vi "CheckDeviceFCG.vi"() -> ()   [LabVIEW 2010]
panel:
  out "WavelenghtArrayOut":i32[](array[numeric])
  out "OnlineStatusLaserPower":bool
  out "Interlock":bool
  out "Diode (pump) current / [mA]":i32(knob)=2 scale=0.0..700.0
  out "Booster 1 current / [mA]":i32(knob) scale=0.0..5000.0
  out "Output photodiode current / [mA]":i32(knob) scale=0.0..200.0
  out "Actual Power Level / [%]":i8(knob) scale=0.0..100.0
  out "Temperature sensor 1 / [°C]":i8(knob)=24 scale=20.0..30.0
  out "Temperature sensor 3 / [°C]":i8(knob)=25 scale=20.0..30.0
  out "Temperature sensor 2 / [°C]":i8(knob)=24 scale=20.0..30.0
  out "Temperature sensor 0 / [°C]":i8(knob)=23 scale=20.0..30.0
  out "andorscanner":bool
  out "710 Get":bool
  out "517 Get":bool
  out "ctiotf Get":bool
  out "Camera Get":bool
  out "Seed Laser Get":bool caption="seed laser"
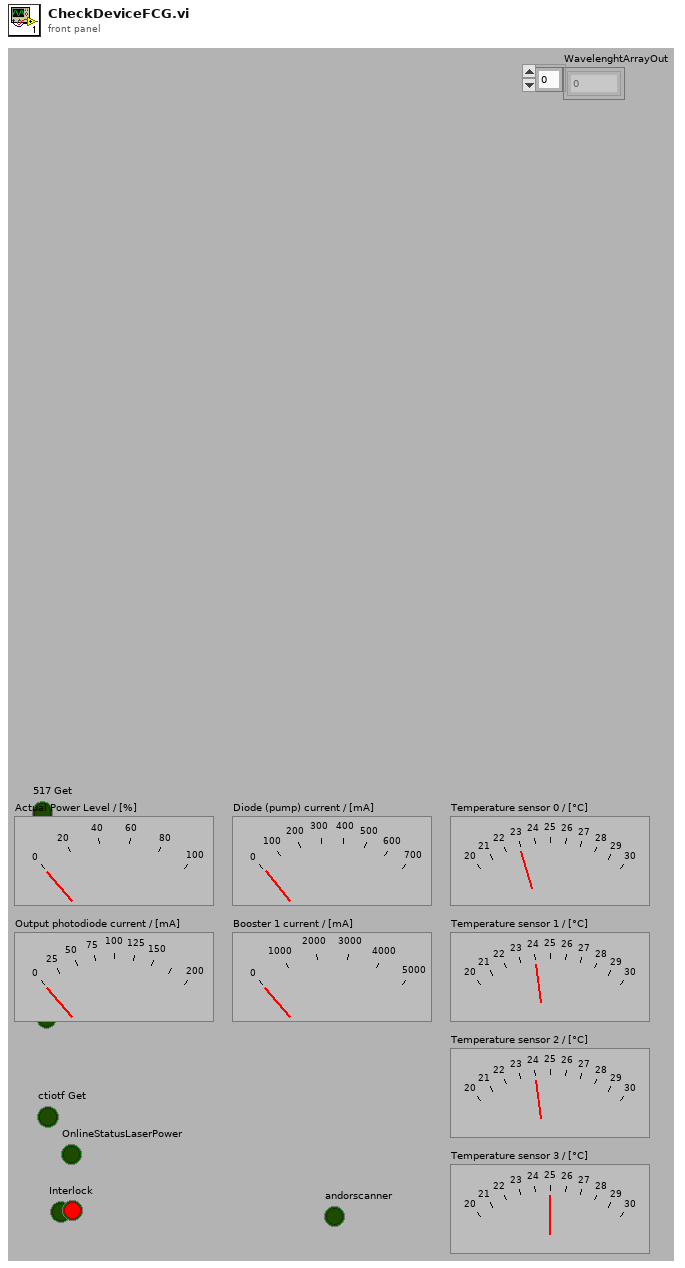
[diagram p1: front panel]
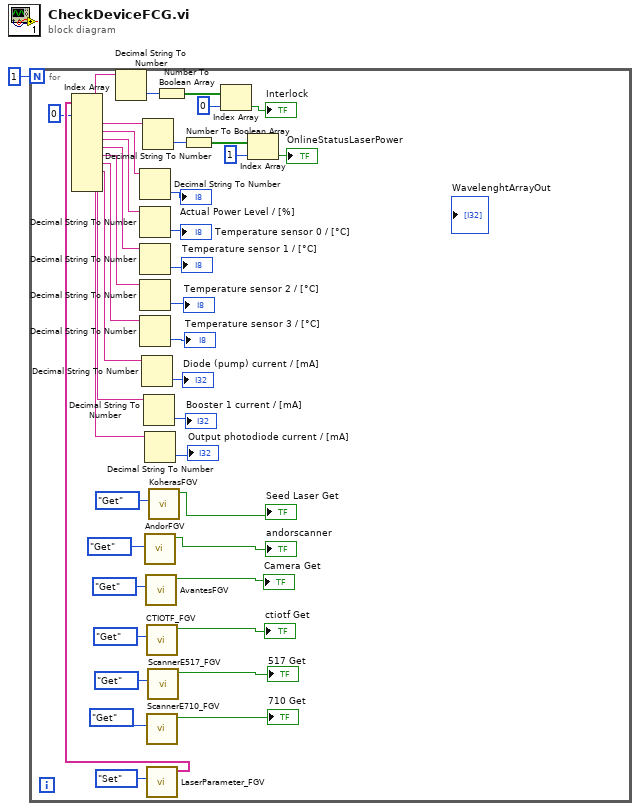
[diagram p0: block diagram]
diagram:
  n1 = for {
    N: 1 -> [_]
    n2 = call "AndorFGV.vi"("Set_Get"=enum16{"Set", "Get"}."Get") -> ("andor 0"=→"andorscanner":bool)  [unwired: 8 in, 2 out]
    n3 = call "AvantesFGV.vi"("Set_Get"=enum16{"Set", "Get"}."Get") -> ("Get"=→"Camera Get":bool)  [unwired: 9 in, 1 out]
    n4 = call "CTIOTF_FGV.vi"("Set_Get"=enum16{"Set", "Get"}."Get") -> ("aotfGet"=→"ctiotf Get":bool)  [unwired: 9 in, 1 out]
    n5 = call "ScannerE710_FGV.vi"("Set_Get"=enum16{"Set", "Get"}."Get") -> ("Get"=→"710 Get":bool)  [unwired: 9 in, 1 out]
    n6 = call "LaserParameter_FGV.vi"("Set_Get"=enum16{"Set", "Get"}."Set") -> ("LaserParameterGet"=w5:string[])  [unwired: 9 in, 1 out]
    n7 = Index Array(array=w5, index #1=0 ("index")) -> (element #1=w21:string, element #2=w20:string, element #3=w19:string, element #4=w18:string, element #5=w11:string, element #6=w10:string, element #7=w9:string, element #8=w8:string, element #9=w7:string, element #10=w6:string)  [unwired: 9 in]
    n8 = Decimal String To Number(string=w21) -> (number=w17:i32)  [unwired: 2 in, 1 out]
    n9 = Decimal String To Number(string=w19) -> (number=→"Actual Power Level / [%]":i32)  [unwired: 2 in, 1 out]
    n10 = Decimal String To Number(string=w18) -> (number=→"Temperature sensor 0 / [°C]":i32)  [unwired: 2 in, 1 out]
    n11 = Decimal String To Number(string=w11) -> (number=→"Temperature sensor 1 / [°C]":i32)  [unwired: 2 in, 1 out]
    n12 = Decimal String To Number(string=w10) -> (number=→"Temperature sensor 2 / [°C]":i32)  [unwired: 2 in, 1 out]
    n13 = Decimal String To Number(string=w9) -> (number=→"Temperature sensor 3 / [°C]":i32)  [unwired: 2 in, 1 out]
    n14 = Decimal String To Number(string=w8) -> (number=→"Diode (pump) current / [mA]":i32)  [unwired: 2 in, 1 out]
    n15 = Decimal String To Number(string=w20) -> (number=w16:i32)  [unwired: 2 in, 1 out]
    n16 = Decimal String To Number(string=w7) -> (number=→"Booster 1 current / [mA]":i32)  [unwired: 2 in, 1 out]
    n17 = Decimal String To Number(string=w6) -> (number=→"Output photodiode current / [mA]":i32)  [unwired: 2 in, 1 out]
    n18 = call "ScannerE517_FGV.vi"("Set_Get"=enum16{"Set", "Get"}."Get") -> ("Get"=→"517 Get":bool)  [unwired: 9 in, 1 out]
    n19 = call "KoherasFGV.vi"("Set_Get"=enum16{"Set", "Get"}."Get") -> ("Get"=→"Seed Laser Get":bool)  [unwired: 9 in, 1 out]
    n20 = Number To Boolean Array(number=w17) -> (Boolean array=w15:bool[])
    n21 = Number To Boolean Array(number=w16) -> (Boolean array=w12:bool[])
    n22 = Index Array(array=w15, index=0) -> (element=→"Interlock":bool)
    n23 = Index Array(array=w12, index=1) -> (element=→"OnlineStatusLaserPower":bool)
  }
